vi "OverlayTrackingInfo.vi"(8 "error in (no error)":errorcluster, 9 "maxDistance":i32, 10 "Ball Tracking Position Data":T2, 11 "Image in":T1) -> (0 "error out":errorcluster, 3 "Processed Image Out":T1)   [LabVIEW 2015]
uses:
  <vilib>/vision/Image Controls.llb/IMAQ Image.ctl
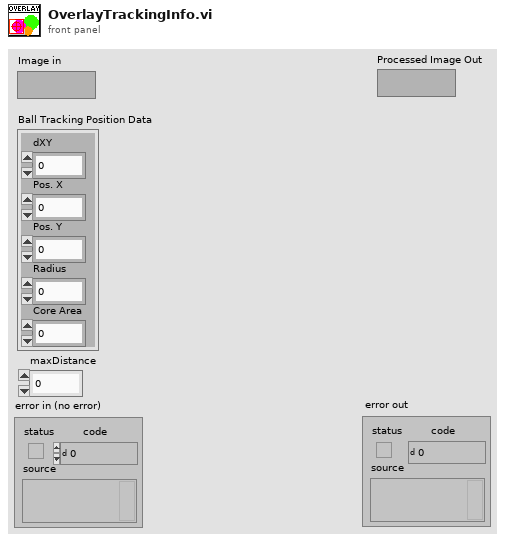
[diagram p1: front panel]
types:
  T1 = typedef "IMAQ Image.ctl" = refnum<image>
  T2 = cluster{"dXY":i32, "Pos. X":i32, "Pos. Y":i32, "Radius":i32, "Core Area":i32}
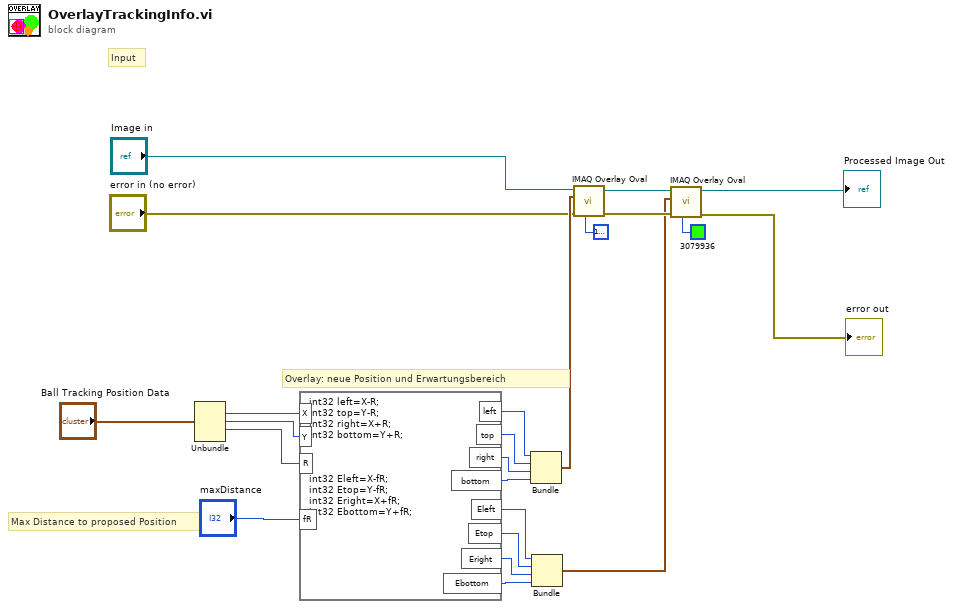
[diagram p0: block diagram]
diagram:
  # "Input"
  # "Max Distance to proposed Position"
  # "Overlay: neue Position und Erwartungsbereich"
  n1 = Unbundle("Ball Tracking Position Data") -> ("Pos. X"=w18:i32, "Pos. Y"=w17:i32, "Radius"=w16:i32)  [unwired: 2 out]
  n2 = formula code="int32 left=X-R;\nint32 top=Y-R;\nint32 right=X+R;\nint32 bottom=Y+R;\n\n\n\nint32 Eleft=X-fR;\nint32 Etop=Y-fR;\nint32 Eright=X+fR;\nint32 Ebottom=Y+fR;"("X"=w18, "Y"=w17, "R"=w16, "fR"="maxDistance") -> ("left"=w10:i32, "top"=w23:i32, "right"=w22:i32, "bottom"=w21:i32, "Eleft"=w9:i32, "Etop"=w8:i32, "Eright"=w7:i32, "Ebottom"=w6:i32)
  n3 = Bundle(w10, w23, w22, w21) -> (w19:cluster{i32, i32, i32, i32})  [unwired: 1 in]
  n4 = Bundle(w9, w8, w7, w6) -> (w5:cluster{i32, i32, i32, i32})  [unwired: 1 in]
  n5 = call "IMAQ Overlay Oval"("Color"=u32 16777226, "error in (no error)"="error in (no error)", "Bounding Rectangle"=w19, "Image"="Image in") -> ("error out"=w13:errorcluster, "Image Out"=w15:T1)  [unwired: 6 in]
  n6 = call "IMAQ Overlay Oval"("Color"=u32 3079936, "error in (no error)"=w13, "Bounding Rectangle"=w5, "Image"=w15) -> ("error out"=→"error out":errorcluster, "Image Out"=→"Processed Image Out":T1)  [unwired: 6 in]
